vi "table_to_array.vi"(6 "usuario_registra":i32, 8 "error in (no error)":errorcluster, 9 "Tabla Referencia Acústica Generador Externo":string[][](array[string]), 10 "id_pon_frecuencia":i32, 11 "last_id_ajuste_previo":string) -> (0 "error out":errorcluster, 3 "Array":string[](array[string]))   [LabVIEW 2019, in "Base de Datos.lvclass"]
uses:
  Base de Datos.lvclass
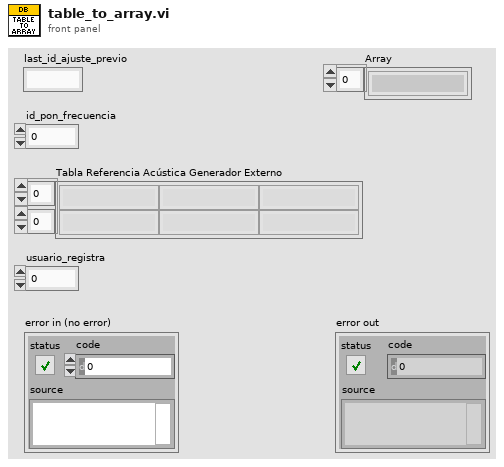
[diagram p1: front panel]
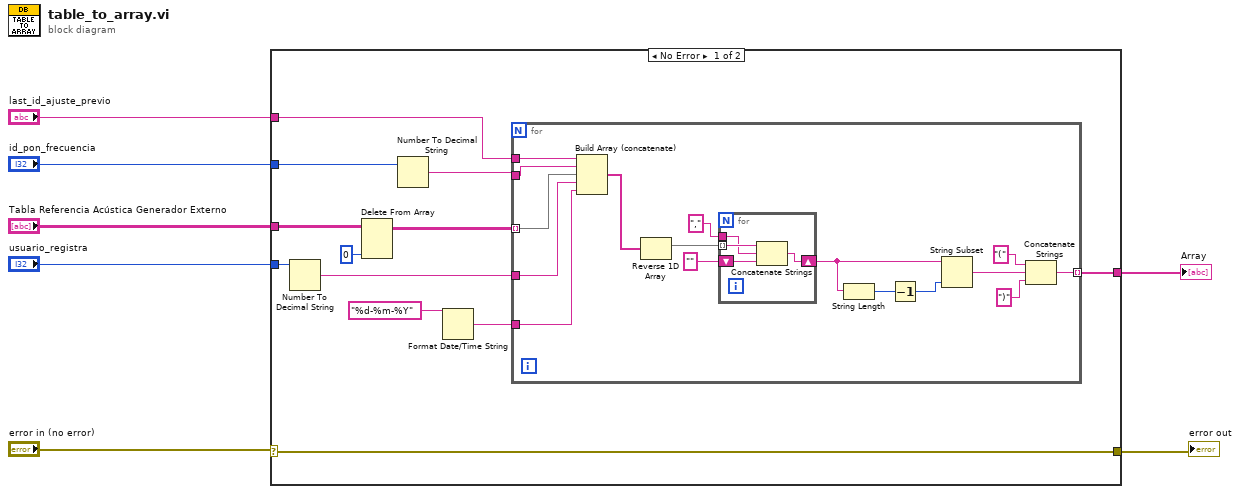
[diagram p0: block diagram]
diagram:
  n1 = case shown="No Error" "error in (no error)" {
    selector: "error in (no error)" -> [w9 w40]
    tunnel: "usuario_registra" -> [w18 _]
    tunnel: "id_pon_frecuencia" -> [w17 _]
    tunnel: [w15 _] -> w5
    tunnel: "Tabla Referencia Acústica Generador Externo" -> [w14 _]
    tunnel: "last_id_ajuste_previo" -> [w8 _]
    tunnel: [w9 w40] -> w1
    frame No Error {
      n2 = Number To Decimal String(number=w18) -> (decimal integer string=w19:string)  [unwired: 1 in]
      n3 = Delete From Array(array=w14, index (col)=0 ("disabled index (col)")) -> (array with subset deleted=w13:string[][])  [unwired: 2 in, 1 out]
      n4 = Number To Decimal String(number=w17) -> (decimal integer string=w16:string)  [unwired: 1 in]
      n5 = Format Date/Time String(time format string (%c)="%d-%m-%Y") -> (date/time string=w11:string)  [unwired: 2 in]
      n6 = for {
        tunnel: w16 -> [w35]
        tunnel: w19 -> [w34]
        tunnel: w11 -> [w33]
        tunnel: w13 -> [w26] mode=indexing
        tunnel: [w24] -> w15 mode=indexing
        tunnel: w8 -> [w20]
        n7 = Build Array (concatenate)(w20, w35, w26, w34, w33) -> (w31:string[])
        n8 = Reverse 1D Array(array=w31) -> (reversed array=w30:string[])
        n9 = for {
          shift-right: [w39] -> w29
          shift-left: "" -> [w38]
          tunnel: w30 -> [w37] mode=indexing
          tunnel: "," ("string") -> [w36]
          n10 = Concatenate Strings(w37, w36, w38) -> (w39:string)
        }
        n11 = String Length(string=w29) -> (length=w28:i32)
        n12 = Decrement(x=w28) -> (x-1=w27:i32)
        n13 = String Subset(string=w29, length (rest)=w27) -> (substring=w25:string)  [unwired: 1 in]
        n14 = Concatenate Strings("(" ("element"), w25, ")" ("element")) -> (w24:string)
      }
    }
    frame Error {
    }
  }
  "Array" <- w5
  "error out" <- w1
